vi "Not A Host Key.vi"(1 "host key":T1) -> (0 "Not a Host Key?":bool)   [LabVIEW 2017, in "libssh2.lvlib"]
doc: "Returns TRUE if <B>host key</B> is not a host key. Otherwise, FALSE."
uses:
  libssh2.lvlib
  Host Key Refnum.ctl
  Host Key Refnum Data.ctl
  Host Key Database Refnum.ctl
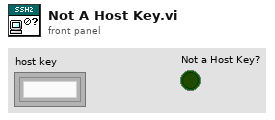
[diagram p1: front panel]
types:
  T1 = typedef "libssh2.lvlib/Host Key Refnum.ctl" = refnum<k1>
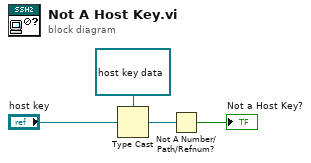
[diagram p0: block diagram]
diagram:
  n1 = Type Cast(type=refnum<data-value> refnum ("data value reference"), x="host key") -> (*(type *) &x=w2:refnum<data-value>)
  n2 = Not A Number/Path/Refnum?(number/path/refnum=w2) -> (NaN/Path/Refnum?=→"Not a Host Key?":bool)
